vi "Write Faulty Meta Data.vi"(6 "options":T3={"ignore timeout error"=TRUE, "timeout ms (1000)"=1000}, 7 "meta data":T2[](array[typedef]), 8 "error in":errorcluster, 11 "connection info in":T1) -> (0 "error out":errorcluster, 3 "connection info out":T1)   [LabVIEW 2013]
doc: "Use this VI to transmit <b>an intentionally faulty</b> meta data cluster to a client. This is useful when developing unit tests."
uses:
  vi.lib/NI/STM/SubVIs/MetaDataElement.ctl
  vi.lib/NI/STM/NI STM.lvlib
  vi.lib/NI/STM/TCP/TCP Connection Info.ctl
  vi.lib/NI/STM/TCP/TCP Write Options.ctl
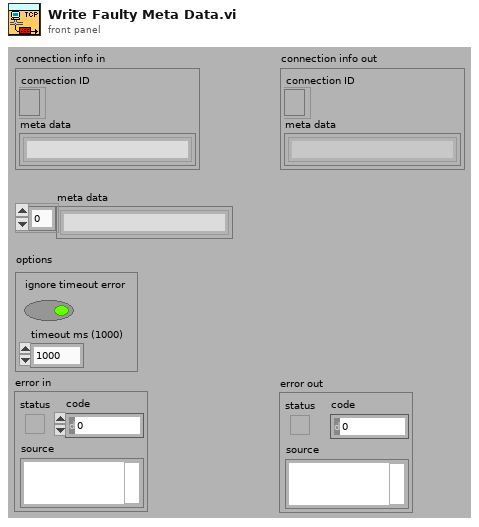
[diagram p1: front panel]
types:
  T1 = typedef "NI STM.lvlib/TCP Connection Info.ctl" = cluster{"connection ID":refnum<k5>, "meta data":T2[]}
  T2 = typedef "NI STM.lvlib/MetaDataElement.ctl" = string
  T3 = typedef "NI STM.lvlib/TCP Write Options.ctl" = cluster{"ignore timeout error":bool, "timeout ms (1000)":i32}
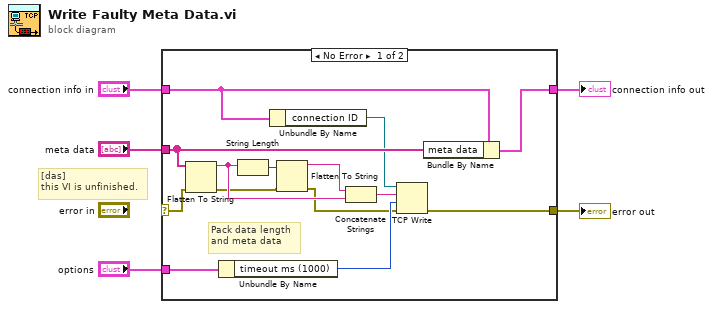
[diagram p0: block diagram]
diagram:
  # "[das]\nthis VI is unfinished."
  n1 = case shown="No Error" {
    selector: _ -> [w10 w21]
    tunnel: [w12 w20] -> w5
    tunnel: "connection info in" -> [w7 w20]
    tunnel: "meta data" -> [w11 _]
    tunnel: [w19 w21] -> w3
    tunnel: "options" -> [w14 _]
    frame No Error {
      # "Pack data length\nand meta data"
      n2 = Flatten To String(anything=w11, error in (no error)=w10) -> (data string=w15:string, error out=w9:errorcluster)  [unwired: 3 out]
      n3 = Unbundle By Name(w14) -> ("timeout ms (1000)"=w13:i32)
      n4 = String Length(string=w15) -> (length=w18:i32)
      n5 = Unbundle By Name(w7) -> ("connection ID"=w6:refnum<k5>)
      n6 = Flatten To String(anything=w18, error in (no error)=w9) -> (data string=w17:string, error out=w8:errorcluster)  [unwired: 3 out]
      n7 = Concatenate Strings(w17, w15) -> (w16:string)
      n8 = TCP Write(connection ID=w6, data in=w16, error in (no error)=w8, 9:w13) -> (error out=w19:errorcluster)  [unwired: 2 out]
      n9 = Bundle By Name(cluster=w7, "meta data"=w11) -> (w12:T1)
    }
    frame Error {
    }
  }
  "connection info out" <- w5
  "error out" <- w3
